vi "Obsługiwanie.vi"(11 "Queue in":refnum<queue>) -> ()   [LabVIEW 2014]
uses:
  Client.ctl
  LukiBrary.lvlib
  Kasy.ctl
panel:
  in  "Kasa":T1
  out "Queue out":refnum<queue>
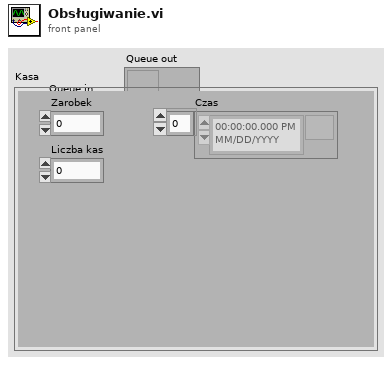
[diagram p1: front panel]
types:
  T1 = typedef "Kasy.ctl" = cluster{"Zarobek":dbl, "Liczba kas":u8, "Czas":timestamp[]}
  T2 = typedef "LukiBrary.lvlib/Client.ctl" = cluster{"Time":dbl, "Price":dbl}
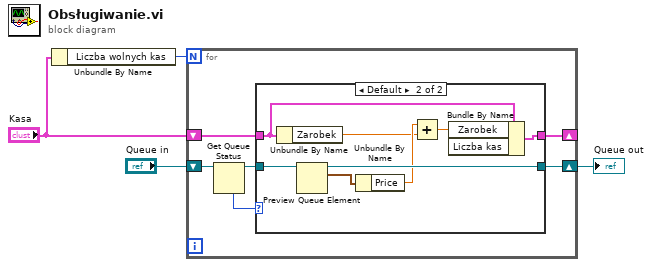
[diagram p0: block diagram]
diagram:
  n1 = Unbundle By Name("Kasa") -> ("Liczba wolnych kas"=w3:u8)
  n2 = for {
    N: w3 -> [_]
    shift-right: [w10] -> w4
    shift-left: "Queue in" -> [w9]
    shift-right: [w5] -> _
    shift-left: "Kasa" -> [w6]
    n3 = Get Queue Status(queue=w9) -> (queue out=w8:refnum<queue>, # elements in queue=w7:i32)  [unwired: 2 in, 6 out]
    n4 = case shown="Default" w7 {
      tunnel: w8 -> [w12 w20]
      tunnel: [w12 w19] -> w10
      tunnel: w6 -> [w11 w15]
      tunnel: [w11 w13] -> w5
      frame 0 {
      }
      frame Default {
        n5 = Unbundle By Name(w15) -> ("Zarobek"=w16:dbl)
        n6 = Preview Queue Element(queue=w20) -> (queue out=w19:refnum<queue>, element=w18:T2)  [unwired: 2 in, 2 out]
        n7 = Unbundle By Name(w18) -> ("Price"=w17:dbl)
        n8 = Add(x=w17, y=w16) -> (x+y=w14:dbl)
        n9 = Bundle By Name(cluster=w15, "Zarobek"=w14) -> (w13:T1)  [unwired: 1 in]
      }
    }
  }
  "Queue out" <- w4
